vi "vacuum practice.vi"() -> ()   [LabVIEW 2018]
uses:
  Classes/Controller/Controller.lvclass
  Classes/Controller/I-O/I-O.lvclass
panel:
  out "Sensor":bool=TRUE
  in  "stop":bool
  in  "Pick up tool vacuum":bool
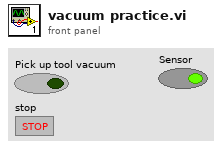
[diagram p1: front panel]
types:
  T1 = typedef "Controller.lvclass/Controllers.ctl" = cluster{"I-O.lvclass":refnum<class "I-O.lvclass">, "Gantry":refnum<k24>, "Dispenser":refnum<visa-resource-name>}
  T2 = typedef "I-O.lvclass/Pin Map.ctl" = cluster{"Region Valves":i32[], "Extra Valves":dbl[][][], "Tool Primary Valve":i32, "Tool Secondary Valve":i32, "Region Sensors":i32[], "Extra Sensors":dbl[][][], "Tool Primary Sensor":dbl, "Tool Secondary Sensor":dbl, "Compression Sensor":dbl, "5V":i32, "Dispenser Sensor":dbl}
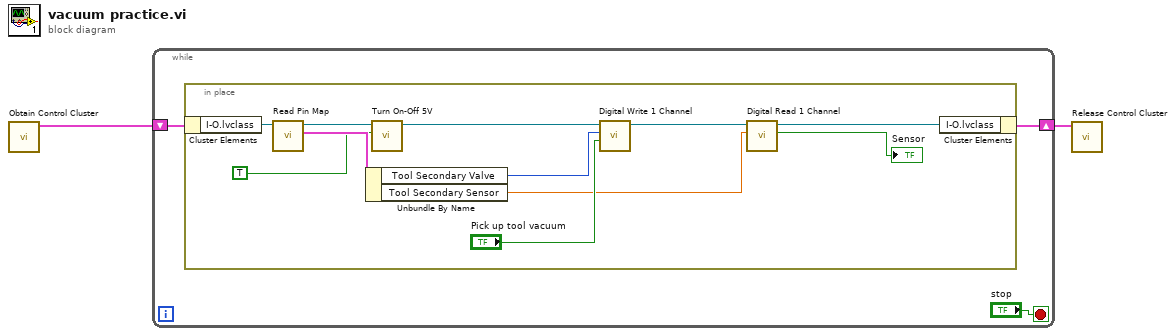
[diagram p0: block diagram]
diagram:
  n1 = call "Obtain Control Cluster.vi"() -> ("Control Out"=w2:T1)  [unwired: 11 in]
  n2 = while {
    shift-right: [w4] -> w1
    shift-left: w2 -> [w5]
    stop <- "stop" stop-if-true
    n3 = in-place {
      n4 = in-place-cluster #1(w5) -> ("I-O.lvclass"=w16:refnum<class "I-O.lvclass">)
      n5 = call-dynamic "Read Pin Map.vi"("I-O in"=w16) -> ("Pin Map 2"=w15:T2, "I-O out"=w8:refnum<class "I-O.lvclass">)  [unwired: 8 in, 1 out]
      n6 = Unbundle By Name(w15) -> ("Tool Secondary Valve"=w14:i32, "Tool Secondary Sensor"=w10:dbl)
      n7 = call-dynamic "Turn On-Off 5V.vi"("Value"=TRUE, "I-O in"=w8) -> ("I-O out"=w7:refnum<class "I-O.lvclass">)  [unwired: 8 in, 1 out]
      n8 = call-dynamic "Digital Write 1 Channel.vi"("Value"="Pick up tool vacuum", "Channel"=w14, "I-O.lvclass"=w7) -> ("I-O.lvclass 2"=w12:refnum<class "I-O.lvclass">)  [unwired: 7 in, 1 out]
      n9 = call-dynamic "Digital Read 1 Channel.vi"("Read"=w10, "I-O in"=w12) -> ("Value"=→"Sensor":bool, "I-O out"=w11:refnum<class "I-O.lvclass">)  [unwired: 7 in, 1 out]
      n10 = in-place-cluster #1("I-O.lvclass"=w11) -> (w4:T1)
    }
  }
  n11 = call "Release Control Cluster.vi"("output cluster"=w1) -> ()  [unwired: 11 in]
